vi "RecursiveSecurityCheck.vi"(8 "error in (no error)":errorcluster, 10 "Blacklist":T1[](array[typedef]), 11 "VI Refnum":refnum<vi>) -> (0 "error out":errorcluster, 1 "Output/Failure":string, 2 "Reject?":bool, 3 "dup VI Refnum":refnum<vi>)   [LabVIEW 2014, in "BuildSecurity.lvlib"]
doc: "Recursively checks the provided VI and any subVIs for blacklisted items. If any item is found, <b>Reject?</b> will return <b>TRUE</b>."
uses:
  BuildSecurity.lvlib
  BlacklistClassInfo.ctl
  <vilib>/Utility/traverseref.llb/TRef TravTarget.ctl
  <vilib>/Utility/traverseref.llb/VI Scripting - Traverse.lvlib
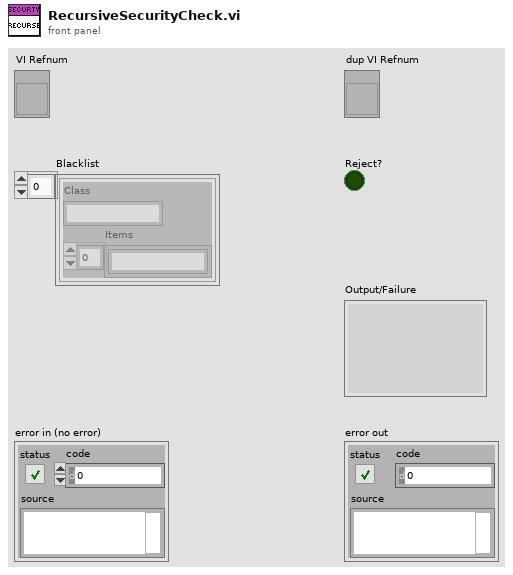
[diagram p1: front panel]
types:
  T1 = typedef "BuildSecurity.lvlib/BlacklistClassInfo.ctl" = cluster{"Class":string, "Items":string[]}
  T2 = enum32{"invalid lock state", "Not Locked", "Locked (No Password)", "Password-protected"}
  T3 = typedef "TRef TravTarget.ctl" = enum16{"FP", "BD", "Other"}
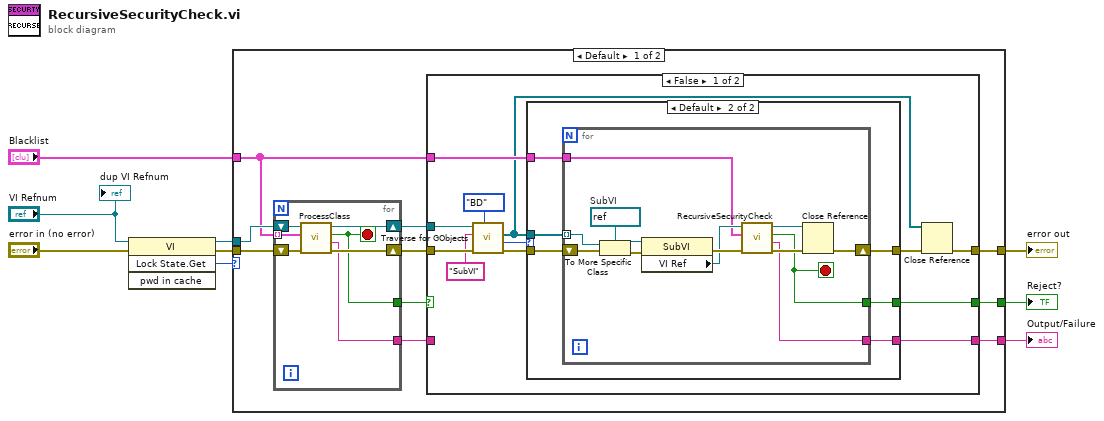
[diagram p0: block diagram]
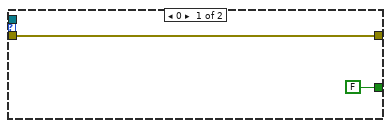
[diagram p2: hidden frame]
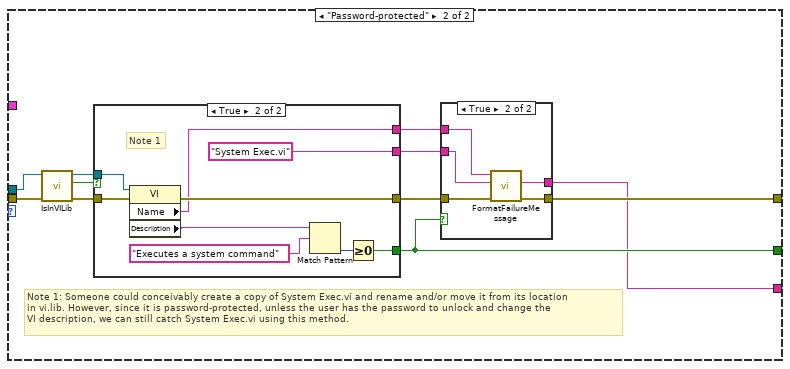
[diagram p4: hidden frame]
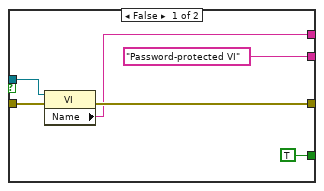
[diagram p6: hidden frame]
diagram:
  n1 = invoke class="VI" method="Lock State.Get"(reference="VI Refnum", error in="error in (no error)") -> (reference out=w5:refnum<vi>, error out=w6:errorcluster, "Get Lock State"=w7:T2)  [unwired: 2 in, 1 out]
  n2 = case shown="Default" w7 {
    tunnel: w6 -> [w19 w73]
    tunnel: w5 -> [w18 w72]
    tunnel: "Blacklist" -> [w12 _]
    tunnel: [w15 w64] -> w3
    tunnel: [w14 w67] -> w2
    tunnel: [w11 w63] -> w1
    frame Default {
      n3 = for {
        shift-right: [w58] -> w16
        shift-left: w19 -> [w62]
        tunnel: w12 -> [w61] mode=indexing
        shift-right: [w59] -> w13
        shift-left: w18 -> [w60]
        tunnel: [w57] -> w17
        tunnel: [w56] -> w10
        stop <- w57 stop-if-true
        n4 = call "ProcessClass.vi"("error in (no error)"=w62, "Blacklist Class"=w61, "VI Refnum"=w60) -> ("error out"=w58:errorcluster, "Output/Failure"=w56:string, "Reject?"=w57:bool, "dup VI Refnum"=w59:refnum<vi>)  [unwired: 5 in]
      }
      n5 = case shown="False" w17 {
        selector: w17 -> [_ w54]
        tunnel: w16 -> [w31 w55]
        tunnel: [w21 w55] -> w15
        tunnel: [w25 w54] -> w14
        tunnel: w13 -> [w29 _]
        tunnel: w12 -> [w24 _]
        tunnel: [w23 w53] -> w11
        tunnel: w10 -> [_ w53]
        frame False {
          n6 = call <vilib>:"Traverse for GObjects.vi"("Traverse Target"=TRef_TravTarget."BD", "error in (no error)"=w31, "Class Name"="SubVI", "VI Refnum"=w29) -> ("error out"=w26:errorcluster, "# of Refs"=w27:i32, "References"=w20:refnum<vi>[])  [unwired: 4 in, 1 out]
          n7 = case shown="Default" w27 {
            tunnel: w26 -> [w33 w39]
            tunnel: [w33 w37] -> w22
            tunnel: [FALSE w36] -> w25
            tunnel: w24 -> [_ w38]
            tunnel: [_ w35] -> w23
            tunnel: w20 -> [_ w34]
            frame 0 {
            }
            frame Default {
              n8 = for {
                shift-right: [w43] -> w37
                shift-left: w39 -> [w49]
                tunnel: w38 -> [w46]
                tunnel: [w42] -> w36
                tunnel: [w41] -> w35
                tunnel: w34 -> [w40] mode=indexing
                stop <- w42 stop-if-true
                w52 = refnum<vi> refnum  # SubVI
                n9 = To More Specific Class(target class=w52, reference=w40, error in=w49) -> (specific class reference=w50:refnum<vi>, error out=w51:errorcluster)
                n10 = property class="SubVI"(reference=w50, error in=w51) -> (error out=w48:errorcluster, "VI Ref"=w47:refnum<vi>)  [unwired: 1 out]
                n11 = call "RecursiveSecurityCheck.vi"("error in (no error)"=w48, "Blacklist"=w46, "VI Refnum"=w47) -> ("error out"=w45:errorcluster, "Output/Failure"=w41:string, "Reject?"=w42:bool, "dup VI Refnum"=w44:refnum<vi>)  [unwired: 5 in]
                n12 = Close Reference(reference=w44, error in (no error)=w45) -> (error out=w43:errorcluster)
              }
            }
          }
          n13 = Close Reference(reference=w20, error in (no error)=w22) -> (error out=w21:errorcluster)
        }
        frame True {
        }
      }
    }
    frame "Password-protected" {
      # "Note 1: Someone could conceivably create a copy of System Exec.vi and rename and/or move it from its location\nin vi.lib. However, since it is password-protected, unless the user has the password to unlock and change the\nVI description, we can still catch System Exec.vi using this method."
      n14 = call "IsInVILib.vi"("error in (no error)"=w73, "VI Refnum"=w72) -> ("error out"=w71:errorcluster, "In vi.lib?"=w69:bool, "dup VI Refnum"=w70:refnum<vi>)  [unwired: 7 in]
      n15 = case shown="True" w69 {
        tunnel: w71 -> [w85 w94]
        tunnel: [w83 w90] -> w68
        tunnel: w70 -> [w84 w93]
        tunnel: [TRUE w89] -> w67
        tunnel: [w81 w87] -> w65
        tunnel: ["Password-protected VI" "System Exec.vi" ("t")] -> w66
        frame False {
          n16 = property class="VI"(reference=w84, error in=w85) -> (error out=w83:errorcluster, "Name"=w81:string)  [unwired: 1 out]
        }
        frame True {
          # "Note 1"
          n17 = property class="VI"(reference=w93, error in=w94) -> (error out=w90:errorcluster, "Name"=w87:string, "Description"=w88:string)  [unwired: 1 out]
          n18 = Match Pattern(string=w88, regular expression="Executes a system command") -> (offset past match=w92:i32)  [unwired: 1 in, 3 out]
          n19 = Greater Or Equal To 0?(x=w92) -> (x >= 0?=w89:bool)
        }
      }
      n20 = case shown="True" w67 {
        tunnel: w68 -> [w74 w79]
        tunnel: w66 -> [_ w77]
        tunnel: w65 -> [_ w78]
        tunnel: [w74 w76] -> w64
        tunnel: [_ w75] -> w63
        frame False {
        }
        frame True {
          n21 = call "FormatFailureMessage.vi"("error in (no error)"=w79, "Restricted Object"=w77, "VI Name"=w78) -> ("error out"=w76:errorcluster, "Output/Failure"=w75:string)  [unwired: 7 in]
        }
      }
    }
  }
  "error out" <- w3
  "Reject?" <- w2
  "Output/Failure" <- w1
  "dup VI Refnum" <- "VI Refnum"
